vi "ServerPrompt.vi"(0 "AzCam Hostname":string="azcam", 1 "Port":u16=2402) -> (2 "ServerOut":string="tester", 3 "Port Out":u16=2402, 4 "Error":bool)   [LabVIEW 2014]
panel:
  in  "Quit":bool
  in  "Connect":bool
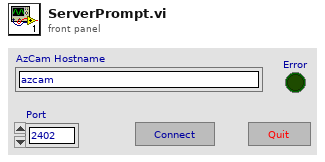
[diagram p1: front panel]
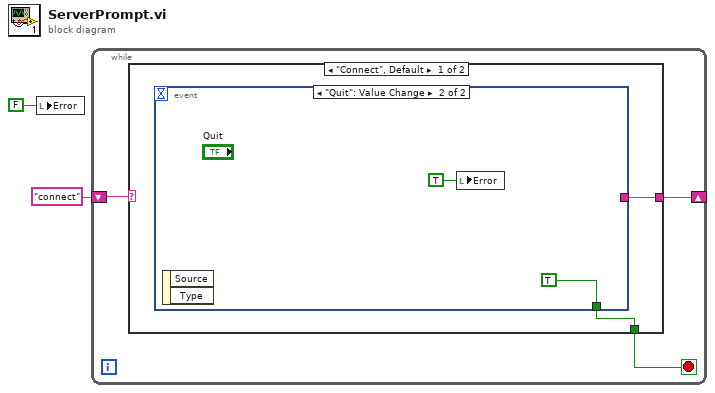
[diagram p0: block diagram]
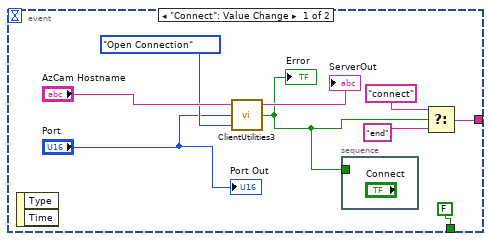
[diagram p2: hidden frame]
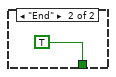
[diagram p3: hidden frame]
diagram:
  n1 = local write "Error"(FALSE ("Error")) -> ()
  n2 = while {
    shift-right: [w4] -> _
    shift-left: "connect" -> [w5]
    stop <- w3 stop-if-true
    n3 = case shown="\"Connect\", Default" w5 {
      tunnel: [w7 _] -> w4
      tunnel: [w6 TRUE] -> w3
      frame "Connect", Default {
        n4 = event shown="[1] \"Quit\": Value Change" {
          selector: _ -> [_ _]
          dyn-events: _ -> [_ _]
          timeout: _ -> [_ _]
          tunnel: [w12 _] -> w7
          tunnel: [FALSE TRUE] -> w6
          event "Connect": Value Change {
            n5 = event-data() -> ()  [unwired: 1 in, 2 out]
            n6 = call "ClientUtilities3.vi"("Action"=enum16{"Open Connection"}."Open Connection", "ServerPort"="Port", "ServerName"="AzCam Hostname") -> ("Error"=w8:bool)
            "Error" <- w8
            n7 = stacked-sequence {
              tunnel: w8 -> [_]
              frame #0 {
              }
            }
            n8 = Select(t="connect", s=w8, f="end") -> (s? t:f=w12:string)
            "ServerOut" <- "AzCam Hostname"
            "Port Out" <- "Port"
          }
          event "Quit": Value Change {
            n9 = event-data() -> ()  [unwired: 1 in, 2 out]
            n10 = local write "Error"(TRUE ("Error")) -> ()
          }
        }
      }
      frame "End" {
      }
    }
  }
